vi "CombineSlow.vi"(1 "HV Cluster":T3={"HV Power On/Off"=[TRUE, TRUE], "Set Voltage(V)"=["0", "0", "0", "0", "0", "0", "0", "0"], "HV Tolerance (%)"=1.0, "Current(uA)"=[]}, 2 "Slow Cluster in":T2) -> (0 "Slow Cluster":T1)   [LabVIEW 2012]
uses:
  hv cluster control.ctl
  Slow cluster control.ctl
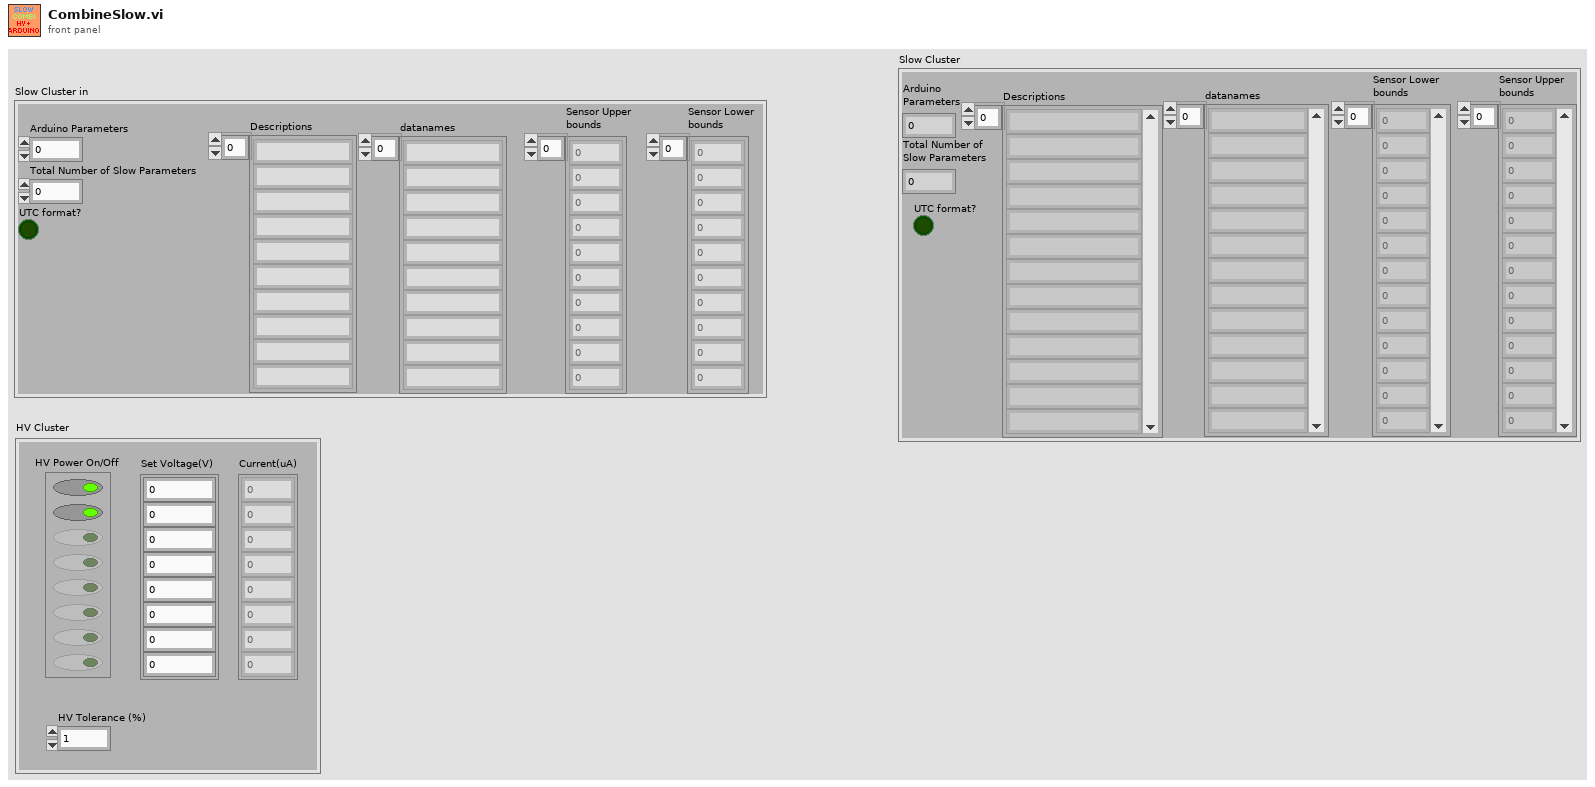
[diagram p1: front panel]
types:
  T1 = typedef "Slow cluster control.ctl" = cluster{"Arduino \nParameters":dbl, "Total Number of \nSlow Parameters":i32, "UTC format?":bool, "Sensor Upper \nbounds":i32[], "Sensor Lower \nbounds":i32[], "Descriptions":string[], "datanames":string[]}
  T2 = cluster{"Arduino Parameters":dbl, "Total Number of Slow Parameters":i32, "UTC format?":bool, "Sensor Upper \nbounds":i32[], "Sensor Lower \nbounds":i32[], "Descriptions":string[], "datanames":string[]}
  T3 = typedef "hv cluster control.ctl" = cluster{"HV Power On/Off":bool[], "Set Voltage(V)":string[], "HV Tolerance (%)":dbl, "Current(uA)":dbl[]}
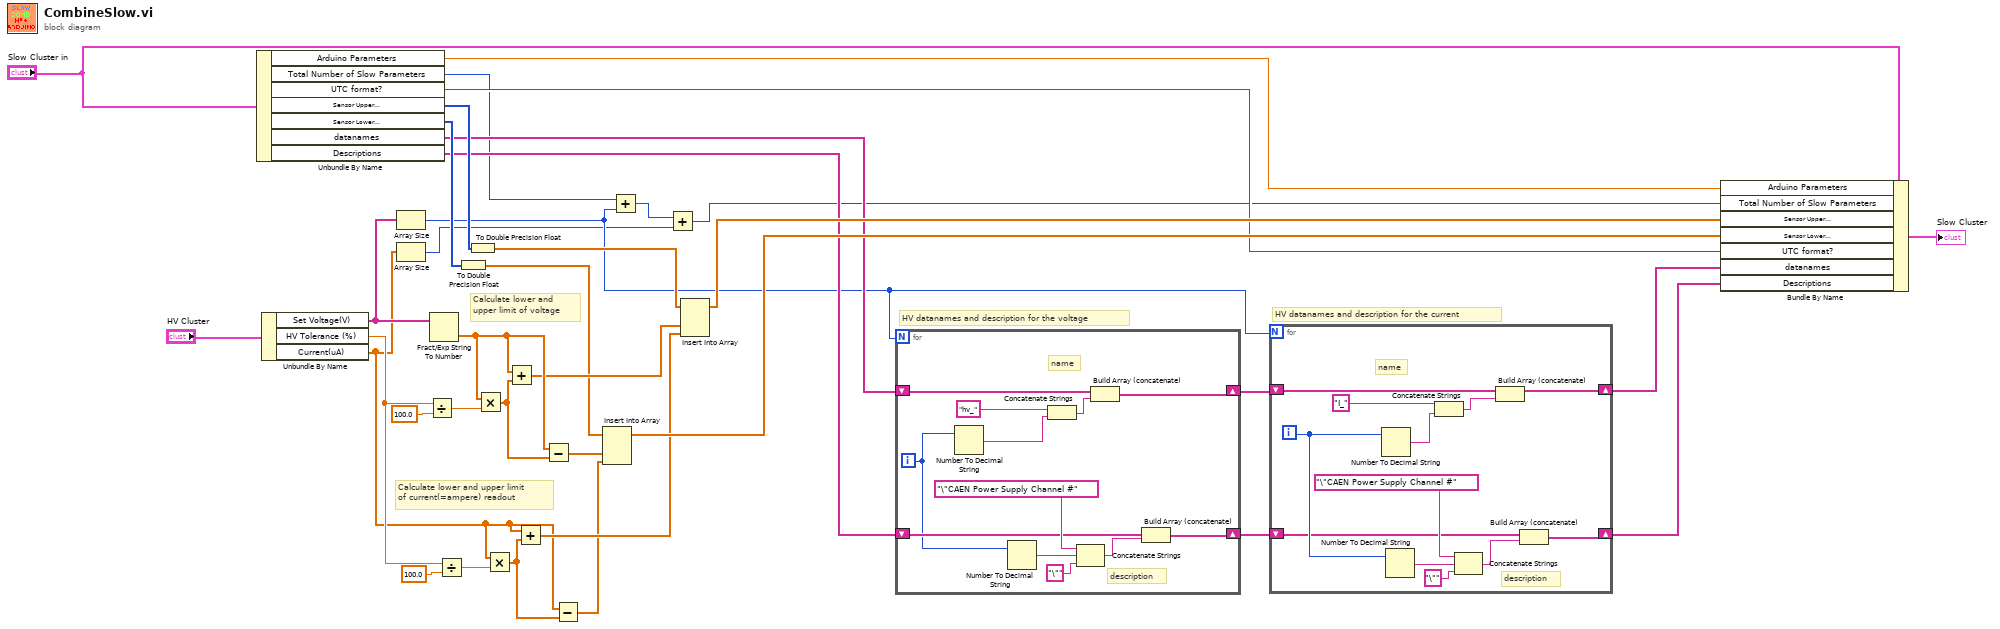
[diagram p0: block diagram]
diagram:
  # "HV datanames and description for the current"
  # "HV datanames and description for the voltage"
  # "Calculate lower and \nupper limit of voltage"
  # "Calculate lower and upper limit\nof current(=ampere) readout"
  n1 = Unbundle By Name("Slow Cluster in") -> ("Arduino Parameters"=w18:dbl, "Total Number of Slow Parameters"=w19:i32, "UTC format?"=w22:bool, "Sensor Upper \nbounds"=w28:i32[], "Sensor Lower \nbounds"=w27:i32[], "datanames"=w21:string[], "Descriptions"=w20:string[])
  n2 = Unbundle By Name("HV Cluster") -> ("Set Voltage(V)"=w25:string[], "HV Tolerance (%)"=w7:dbl, "Current(uA)"=w4:dbl[])
  n3 = Array Size(array=w25) -> (size(s)=w11:i32)
  n4 = Array Size(array=w4) -> (size(s)=w1:i32)
  n5 = Divide(x=w7, y=100.0) -> (x/y=w31:dbl)
  n6 = Fract/Exp String To Number(string=w25) -> (number=w36:dbl[])  [unwired: 3 in, 1 out]
  n7 = Divide(x=w7, y=100.0) -> (x/y=w10:dbl)
  n8 = To Double Precision Float(number=w27) -> (double precision float=w29:dbl[])
  n9 = To Double Precision Float(number=w28) -> (double precision float=w30:dbl[])
  n10 = Multiply(x=w36, y=w31) -> (x*y=w35:dbl[])
  n11 = Multiply(x=w4, y=w10) -> (x*y=w8:dbl[])
  n12 = Add(x=w36, y=w35) -> (x+y=w34:dbl[])
  n13 = Add(x=w4, y=w8) -> (x+y=w6:dbl[])
  n14 = Subtract(x=w36, y=w35) -> (x-y=w33:dbl[])
  n15 = Subtract(x=w4, y=w8) -> (x-y=w5:dbl[])
  n16 = Insert Into Array(array=w29, new element #1=w33, new element #2=w5) -> (w23:dbl[])  [unwired: 1 in]
  n17 = Add(x=w19, y=w11) -> (x+y=w3:i32)
  n18 = Add(x=w3, y=w1) -> (x+y=w2:i32)
  n19 = Insert Into Array(array=w30, new element #1=w34, new element #2=w6) -> (w24:dbl[])  [unwired: 1 in]
  n20 = for {
    N: w11 -> [_]
    shift-right: [w37] -> w14
    shift-left: w21 -> [w44]
    shift-right: [w40] -> w13
    shift-left: w20 -> [w42]
    i -> [w39]
    # "description"
    # "name"
    n21 = Number To Decimal String(number=w39) -> (decimal integer string=w47:string)  [unwired: 1 in]
    n22 = Number To Decimal String(number=w39) -> (decimal integer string=w45:string)  [unwired: 1 in]
    n23 = Concatenate Strings("hv_", w47) -> (w43:string)
    n24 = Concatenate Strings("\"CAEN Power Supply Channel #", w45, "\"" ("element")) -> (w41:string)
    n25 = Build Array (concatenate)(w44, w43) -> (w37:string[])
    n26 = Build Array (concatenate)(w42, w41) -> (w40:string[])
  }
  n27 = for {
    N: w11 -> [_]
    shift-right: [w52] -> w15
    shift-left: w14 -> [w53]
    shift-right: [w49] -> w12
    shift-left: w13 -> [w50]
    i -> [w51]
    # "description"
    # "name"
    n28 = Number To Decimal String(number=w51) -> (decimal integer string=w55:string)  [unwired: 1 in]
    n29 = Number To Decimal String(number=w51) -> (decimal integer string=w57:string)  [unwired: 1 in]
    n30 = Concatenate Strings("I_", w55) -> (w58:string)
    n31 = Concatenate Strings("\"CAEN Power Supply Channel #", w57, "\"" ("element")) -> (w59:string)
    n32 = Build Array (concatenate)(w53, w58) -> (w52:string[])
    n33 = Build Array (concatenate)(w50, w59) -> (w49:string[])
  }
  n34 = Bundle By Name(cluster="Slow Cluster in", "Arduino Parameters"=w18, "Total Number of Slow Parameters"=w2, "Sensor Upper \nbounds"=w24, "Sensor Lower \nbounds"=w23, "UTC format?"=w22, "datanames"=w15, "Descriptions"=w12) -> (→"Slow Cluster":T2)
